vi "Check Amount of Unread Data.vi"(8 "Decrement":bool, 11 "Current Num Points Unread":u16) -> (0 "NumPoinst!=0 before update":bool, 3 "Updated NumPoints Unread":u16)   [LabVIEW 2012]
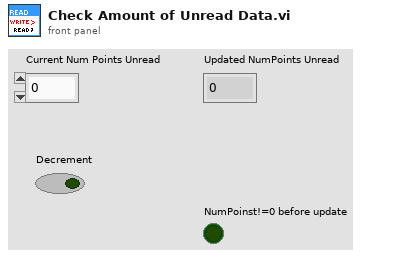
[diagram p1: front panel]
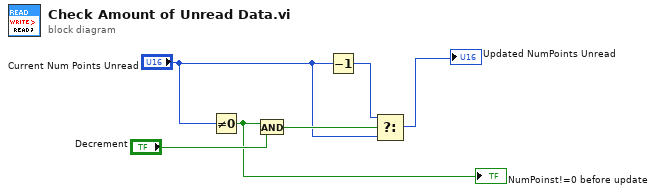
[diagram p0: block diagram]
diagram:
  n1 = Not Equal To 0?(x="Current Num Points Unread") -> (x != 0?=w4:bool)
  "NumPoinst!=0 before update" <- w4
  n2 = And(x=w4, y="Decrement") -> (x .and. y?=w5:bool)
  n3 = Decrement(x="Current Num Points Unread") -> (x-1=w2:u16)
  n4 = Select(t=w2, s=w5, f="Current Num Points Unread") -> (s? t:f=→"Updated NumPoints Unread":u16)
